vi "Board Listing.vi"(8 "error in":errorcluster, 10 "desired port":string) -> (0 "error out":errorcluster, 2 "Array":string[][](array[string]), 3 "Arduino":T1)   [LabVIEW 2020]
uses:
  ArduinoCtrl.ctl
  9c1b3983-c7ab-5c40-aa67-b4885e2fcccb.vi
  <vilib>/Comparison/Equal/Equal Functor/Equal Functor.lvclass
panel:
  out "standard error":string
  out "Table Control":string[][](table)
  out "String":string
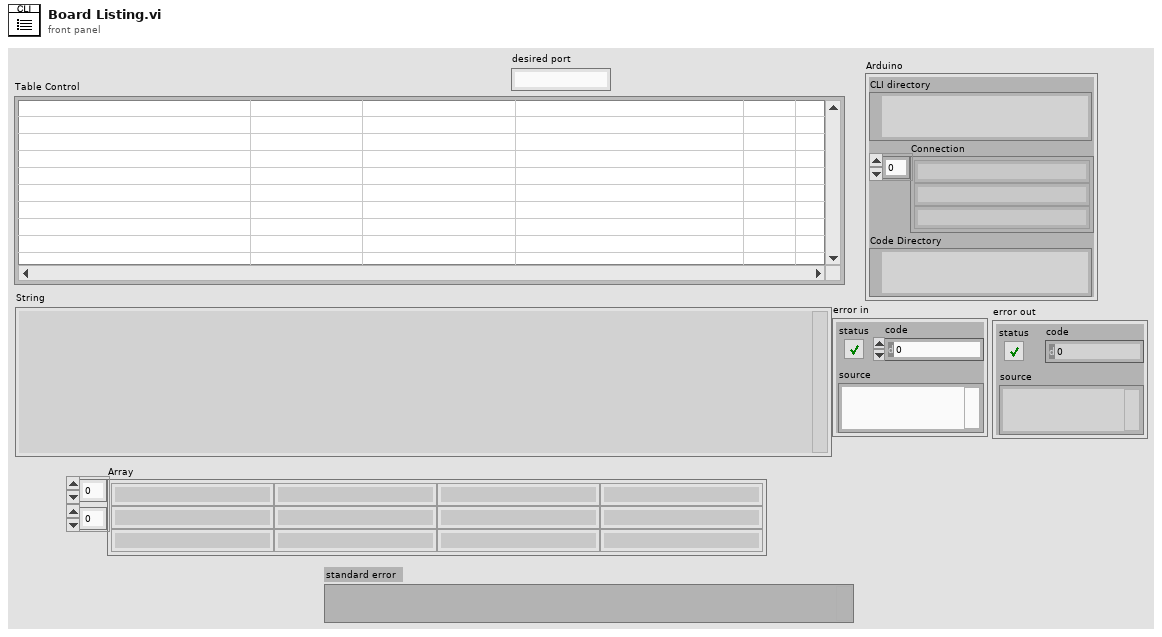
[diagram p1: front panel]
types:
  T1 = typedef "ArduinoCtrl.ctl" = cluster{"CLI directory":path, "Connection":string[], "Code Directory":path}
  T2 = typedef "Preferences.ctl" = cluster{"python":string, "arduino CLI":path, "pythonCodes":cluster{"pythonCode":path, "Color":u32}[], "FontSize":u8, "Text Colors":cluster{"Quote":u32, "function":u32, "Python":u32, "Comment":u32, "Triple Quote":u32, "Text":u32}, "Raspberry Pi":cluster{"Username":string, "password":string}}
  T3 = cluster{"arduino CLI":path, string[], "appended path":path}
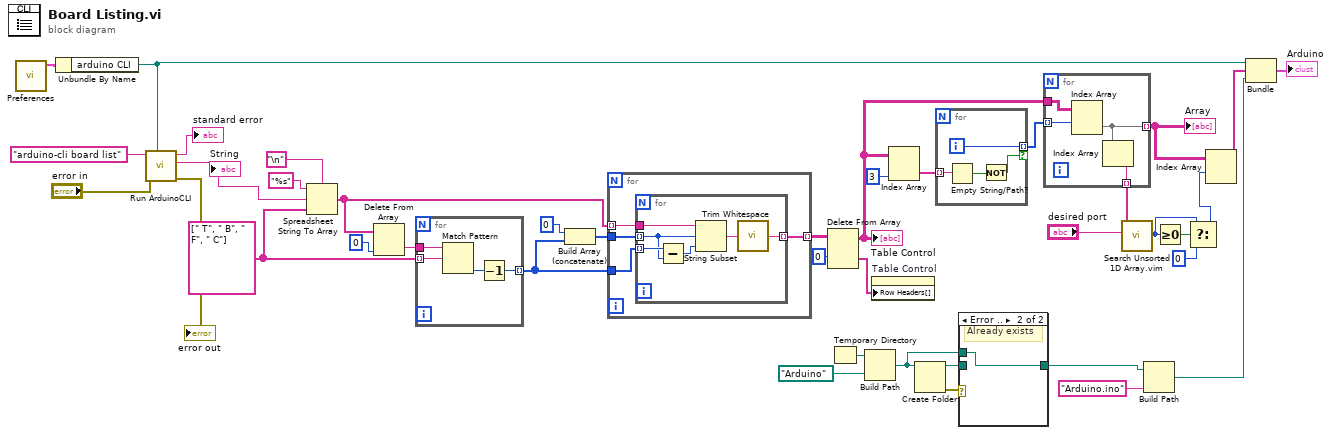
[diagram p0: block diagram]
diagram:
  w36 = string[] [" T", " B", " F", " C"] ("Table Control")
  n1 = call "Preferences.vi"() -> ("Preferences out"=w8:T2)  [unwired: 10 in, 1 out]
  n2 = Unbundle By Name(w8) -> ("arduino CLI"=w7:path)
  n3 = call "Run ArduinoCLI.vi"("working directory"=w7, "error in"="error in", "command line"="arduino-cli board list") -> ("error out"=→"error out":errorcluster, "standard output"=w23:string, "standard error"=→"standard error":string)  [unwired: 6 in]
  "String" <- w23
  n4 = Spreadsheet String To Array(delimiter (Tab)="\n", format string="%s", spreadsheet string=w23, array type (2D Dbl)=w36) -> (array=w31:string[])
  n5 = Delete From Array(array=w31, index=0) -> (deleted portion=w37:string)  [unwired: 1 in, 1 out]
  n6 = for {
    tunnel: w37 -> [w44]
    tunnel: w36 -> [w43] mode=indexing
    tunnel: [w41] -> w34 mode=indexing
    n7 = Match Pattern(string=w44, regular expression=w43) -> (offset past match=w42:i32)  [unwired: 1 in, 3 out]
    n8 = Decrement(x=w42) -> (x-1=w41:i32)
  }
  n9 = Build Array (concatenate)(0, w34) -> (w32:i32[])
  n10 = for {
    tunnel: w31 -> [w48] mode=indexing
    tunnel: w34 -> [w47]
    tunnel: [w46] -> w35 mode=indexing
    tunnel: w32 -> [w45]
    n11 = for {
      tunnel: w48 -> [w54]
      tunnel: w47 -> [w51] mode=indexing
      tunnel: [w49] -> w46 mode=indexing
      tunnel: w45 -> [w50] mode=indexing
      n12 = Subtract(x=w51, y=w50) -> (x-y=w52:i32)
      n13 = String Subset(string=w54, offset (0)=w50, length (rest)=w52) -> (substring=w53:string)
      n14 = call <vilib>:"Trim Whitespace.vi"("string"=w53) -> ("trimmed string"=w49:string)  [unwired: 1 in]
    }
  }
  n15 = Delete From Array(array=w35, index (row)=0) -> (deleted portion=w30:string[], array with subset deleted=w27:string[][])  [unwired: 2 in]
  "Table Control" <- w27
  n16 = Temporary Directory() -> (w6:path)
  n17 = Build Path(base path=w6, name or relative path=path "Arduino") -> (appended path=w1:path)
  n18 = property on="Table Control" class="Tbl (strict)"("Row Headers[]"=w30) -> ()  [unwired: 2 in, 2 out]
  n19 = Index Array(array=w27, index (col)=3 ("disabled index (col)")) -> (element=w28:string[])  [unwired: 1 in]
  n20 = Create Folder(path (use dialog)=w1) -> (created path=w2:path, error out=w4:errorcluster)  [unwired: 2 in, 1 out]
  n21 = for {
    tunnel: w28 -> [w58] mode=indexing
    tunnel: [w57] -> w26 mode=indexing if=w55
    i -> [w57]
    n22 = Empty String/Path?(string/path=w58) -> (empty?=w56:bool)
    n23 = Not(x=w56) -> (.not. x?=w55:bool)
  }
  n24 = case shown="Error .." w4 {
    tunnel: [w59 w60] -> w3
    tunnel: w2 -> [w59 _]
    tunnel: w1 -> [_ w60]
    frame No Error {
    }
    frame Error {
      # "Already exists"
    }
  }
  n25 = for {
    tunnel: w27 -> [w64]
    tunnel: w26 -> [w63] mode=indexing
    tunnel: [w62] -> w21 mode=indexing
    tunnel: [w61] -> w14 mode=indexing
    n26 = Index Array(array=w64, index (row)=w63) -> (element=w62:string[])  [unwired: 1 in]
    n27 = Index Array(array=w62) -> (element=w61:string)  [unwired: 1 in]
  }
  "Array" <- w21
  n28 = call "Search Unsorted 1D Array.vim"("element"="desired port", "unsorted 1D array"=w14) -> ("index of element"=w11:i32)  [unwired: 9 in]
  n29 = Build Path(base path=w3, name or relative path="Arduino.ino") -> (appended path=w17:path)
  n30 = Greater Or Equal To 0?(x=w11) -> (x >= 0?=w12:bool)
  n31 = Select(t=w11, s=w12, f=0) -> (s? t:f=w9:i32)
  n32 = Index Array(array=w21, index (row)=w9) -> (element=w20:string[])  [unwired: 1 in]
  n33 = Bundle("arduino CLI"=w7, w20, "appended path"=w17) -> (→"Arduino":T3)  [unwired: 1 in]
